vi "latch till ready for input.vi"(6 "Ready for Output":bool, 11 "Request Valid":bool) -> (3 "output valid":bool)   [LabVIEW 2023]
uses:
  <instrlib>/_niInstr/Basic Elements/v1/FPGA/niInstr Basic Elements v1 FPGA.lvlib
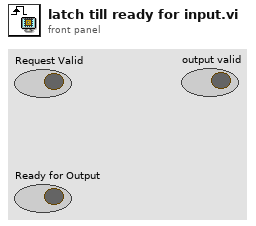
[diagram p1: front panel]
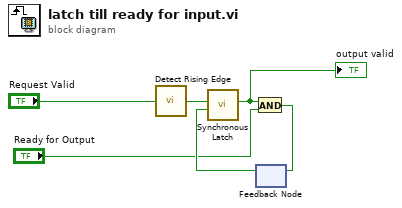
[diagram p0: block diagram]
diagram:
  n1 = call <instrlib>:"Detect Rising Edge.vi"("signal"="Request Valid") -> ("edge detected"=w6:bool)  [unwired: 14 in]
  n2 = feedback #1() -> (w4:bool)  [unwired: 1 in]
  n3 = call <instrlib>:"Synchronous Latch.vi"("clear"=w4, "set"=w6) -> ("out"=w5:bool)  [unwired: 9 in]
  "output valid" <- w5
  n4 = And(x=w5, y="Ready for Output") -> (x .and. y?=w3:bool)
  n5 = feedback-in #1(w3) -> ()
